vi "Font Scale from Required Height.vi"   [LabVIEW 2020, in "g_ar_toolkit.image.lvlib"]
uses:
  g_ar_toolkit.image.lvlib
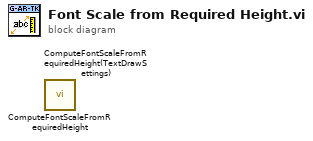
[diagram p0: block diagram]
diagram:
  n1 = call "ComputeFontScaleFromRequiredHeight.vi"() -> ()  [unwired: 10 in, 2 out]
  n2 = call "ComputeFontScaleFromRequiredHeight(TextDrawSettings).vi"() -> ()  [unwired: 10 in, 2 out]
